vi "SD Card.vi"() -> ()   [LabVIEW 2013]
uses:
  <vilib>/FPGAPlugInAG/sbRIO-9626/niLvFpga_Open_sbRIO-9626.vi
  <vilib>/LabVIEW Targets/FPGA/RIO/CompactRIO/cRIO-91xx/cRIO-91XX_MountSdDrive.vi
  <vilib>/rvi/interface/nirviOpenFPGA/nirviOpenFPGA.xnode
  Controls/FPGA_Reference.ctl
  FPGA/bitfiles/TI sbRIO PWM (FPGA) v1.0.lvbitx
  <vilib>/rvi/interface/nirviMethod/nirviMethod.xnode
  <vilib>/LabVIEW Targets/FPGA/RIO/CompactRIO/cRIO-91xx/cRIO-91XX_UnmountSdCardImpl.vi
  <vilib>/LabVIEW Targets/FPGA/RIO/CompactRIO/cRIO-91xx/cRIO-91XX_DirtyMountSdDrive.vi
panel:
  out "Drive Letter 2":path
  out "Drive Handle 2":u32
  out "Drive Letter":path
  out "Drive Handle":u32
  out "error out 4":errorcluster
  out "error out 3":errorcluster
  out "error out 2":errorcluster
  out "path out":path
  out "volume path 2":path
  out "size (bytes)":i64
  out "free (bytes)":i64
  out "error out":errorcluster
  out "volume path":path
  out "stripped path":path
  out "folder names 4":string[](array[string])
  out "dup path":path
  out "file or folder exists?":bool
  out "folder names 3":string[](array[string])
  out "folder names 2":string[](array[string])
  out "folder names":string[](array[string])
  out "filenames":string[](array[string])
  out "path":path
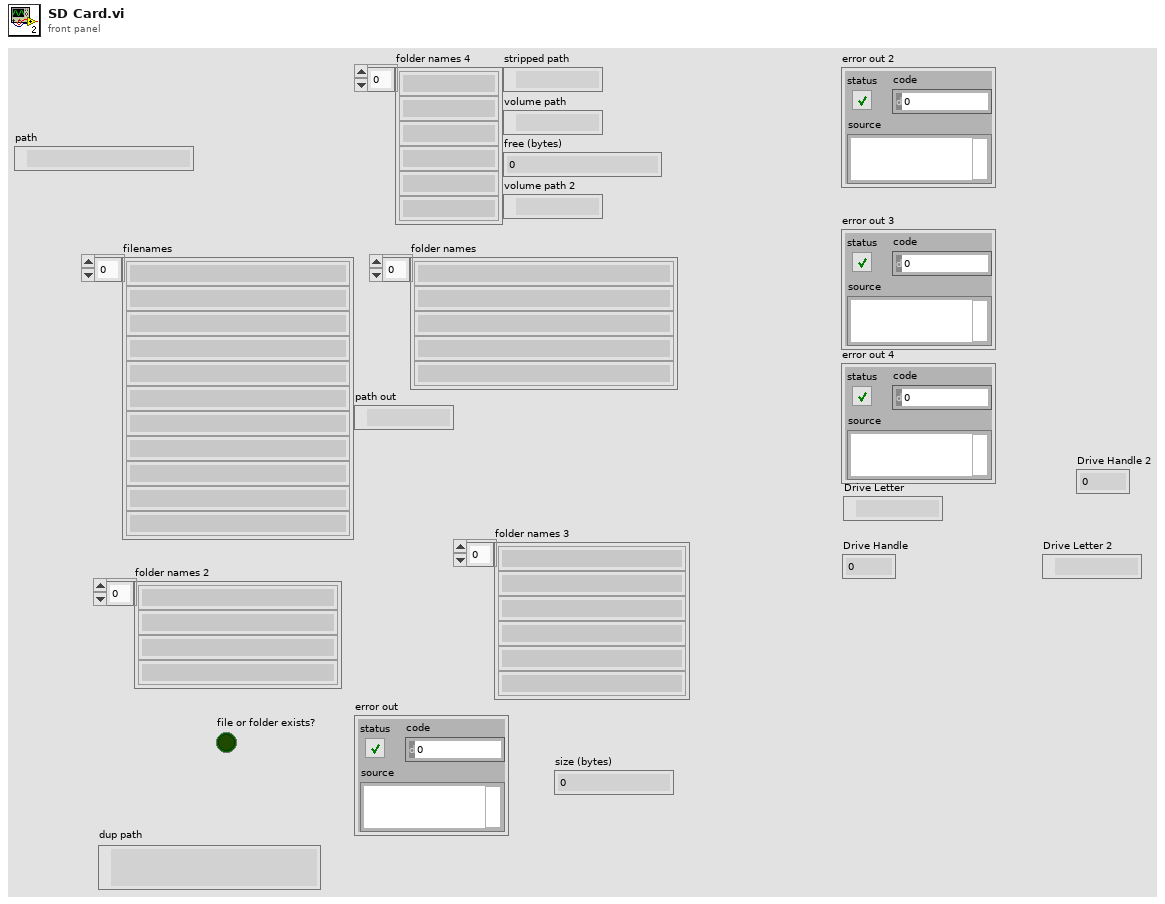
[diagram p1: front panel]
types:
  T1 = typedef "FPGA_Reference.ctl" = refnum<k20>
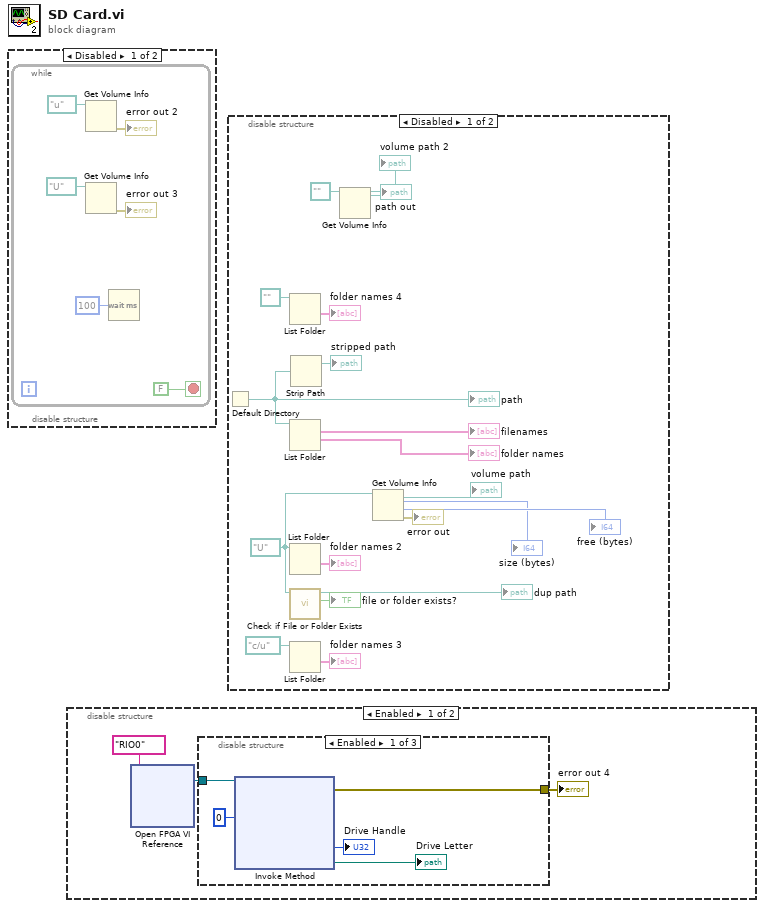
[diagram p0: block diagram]
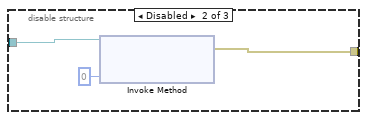
[diagram p4: hidden frame]
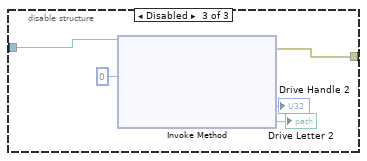
[diagram p5: hidden frame]
diagram:
  n1 = disable-structure shown="Disabled" {
    frame Disabled {
      n2 = while {
        stop <- FALSE stop-if-true
        n3 = Get Volume Info(11:path "u:/" ("path")) -> (0:→"error out 2":errorcluster)  [unwired: 1 in, 5 out]
        n4 = Get Volume Info(11:path "U:/" ("path")) -> (0:→"error out 3":errorcluster)  [unwired: 1 in, 5 out]
        n5 = Wait (ms)(milliseconds to wait=u32 100) -> ()  [unwired: 1 out]
      }
    }
    frame Enabled {
    }
  }
  n6 = disable-structure shown="Enabled" {
    frame Enabled {
      n7 = xnode "Open FPGA VI Reference"("resource name"=tag "RIO0") -> ("FPGA VI Reference Out"=w8:T1)  [unwired: 1 in, 1 out]
      n8 = disable-structure shown="Enabled" {
        disable-tunnel: w8 -> [w14 w17 w22]
        disable-tunnel: [w12 w16 w21] -> w7
        frame Enabled {
          n9 = xnode "Invoke Method"("FPGA VI Reference In"=w14, "Module"=u8 0) -> ("error out"=w12:errorcluster, "Drive Handle"=→"Drive Handle":u32, "Drive Letter"=→"Drive Letter":path)  [unwired: 2 in, 1 out]
        }
        frame Disabled {
          n10 = xnode "Invoke Method"("FPGA VI Reference In"=w17, "Drive Handle"=u32 0) -> ("error out"=w16:errorcluster)  [unwired: 1 in, 1 out]
        }
        frame Disabled {
          n11 = xnode "Invoke Method"("FPGA VI Reference In"=w22, "Module"=u8 0) -> ("error out"=w21:errorcluster, "Drive Handle"=→"Drive Handle 2":u32, "Drive Letter"=→"Drive Letter 2":path)  [unwired: 2 in, 1 out]
        }
      }
      "error out 4" <- w7
    }
    frame Disabled {
    }
  }
  n12 = disable-structure shown="Disabled" {
    frame Disabled {
      w30 = path "U:/" ("path")
      n13 = Default Directory() -> (w32:path)
      "path" <- w32
      n14 = List Folder(path=path "") -> (folder names=→"folder names 4":string[])  [unwired: 3 in, 3 out]
      n15 = List Folder(path=w32) -> (filenames=→"filenames":string[], folder names=→"folder names":string[])  [unwired: 3 in, 2 out]
      n16 = List Folder(path=w30) -> (folder names=→"folder names 2":string[])  [unwired: 3 in, 3 out]
      n17 = call <vilib>:"Check if File or Folder Exists.vi"("path"=w30) -> ("file or folder exists?"=→"file or folder exists?":bool, "dup path"=→"dup path":path)  [unwired: 8 in, 1 out]
      n18 = List Folder(path=path "c:/u") -> (folder names=→"folder names 3":string[])  [unwired: 3 in, 3 out]
      n19 = Strip Path(path=w32) -> (stripped path=→"stripped path":path)  [unwired: 1 out]
      n20 = Get Volume Info(11:path "" ("path")) -> (3:→"path out":path, 5:→"volume path 2":path)  [unwired: 1 in, 4 out]
      n21 = Get Volume Info(11:w30) -> (0:→"error out":errorcluster, 1:→"free (bytes)":i64, 2:→"size (bytes)":i64, 5:→"volume path":path)  [unwired: 1 in, 2 out]
    }
    frame Enabled {
    }
  }
